vi "NET_Sensitivity.vi"(8 "Read(F) Write(T)":bool, 11 "Sen In":T1) -> (3 "Sen  Out":T1)   [LabVIEW 2017]
uses:
  RoboRio Code/TypeDef/CLUSTER_Sensitivities.ctl
  <vilib>/Rock Robotics/Network Tables/NT Read Numeric Array.vi
  <vilib>/Rock Robotics/Network Tables/NT Write Numeric Array.vi
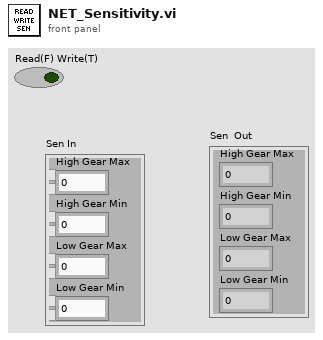
[diagram p1: front panel]
types:
  T1 = typedef "CLUSTER_Sensitivities.ctl" = cluster{"High Gear Max":dbl, "High Gear Min":dbl, "Low Gear Max":dbl, "Low Gear Min":dbl}
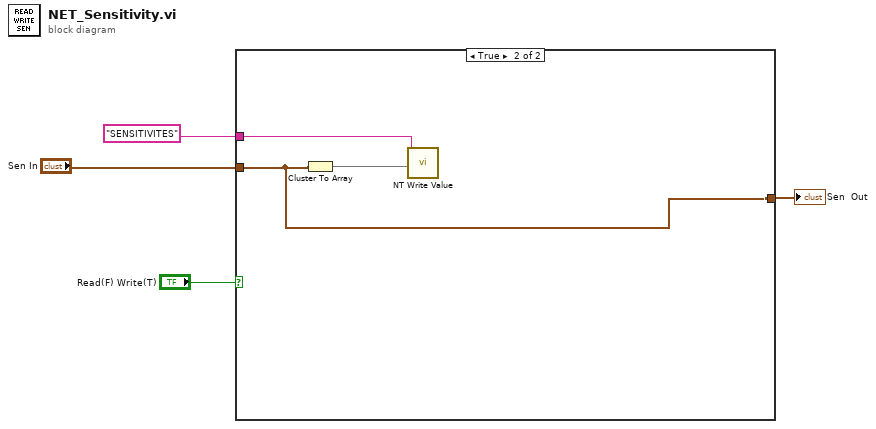
[diagram p0: block diagram]
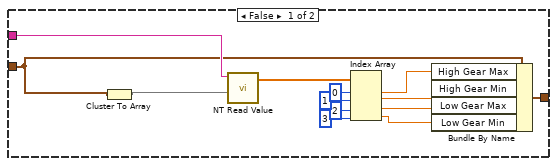
[diagram p2: hidden frame]
diagram:
  n1 = case shown="True" "Read(F) Write(T)" {
    tunnel: "SENSITIVITES" ("Name") -> [w17 w20]
    tunnel: "Sen In" -> [w11 w18]
    tunnel: [w9 w18] -> w2
    frame False {
      n2 = Cluster To Array(cluster=w11) -> (array=w10:dbl[])
      n3 = call-poly <vilib>:"NT Read Value.vi"("Default Value"=w10, "Name"=w17) -> ("Numeric Array"=w16:dbl[])  [unwired: 8 in, 1 out]
      n4 = Index Array(array=w16, index #1=0 ("index"), index #2=1 ("index"), index #3=2 ("index"), index #4=3 ("index")) -> (element #1=w8:dbl, element #2=w7:dbl, element #3=w6:dbl, element #4=w5:dbl)
      n5 = Bundle By Name(cluster=w11, "High Gear Max"=w8, "High Gear Min"=w7, "Low Gear Max"=w6, "Low Gear Min"=w5) -> (w9:T1)
    }
    frame True {
      n6 = Cluster To Array(cluster=w18) -> (array=w19:dbl[])
      n7 = call-poly <vilib>:"NT Write Value.vi"("Numeric Array"=w19, "Name"=w20) -> ()  [unwired: 9 in, 1 out]
    }
  }
  "Sen  Out" <- w2
